vi "get 2d spectrum data.vi"(6 "data in":T5={"Total counts"=0, "cps"=0.0, "live time"=0.0, "pulser"=0.0, "rare counts"=0.0, "other counts"=0.0, "total run time(sec)"=0.0, "adjusted run time(sec)"=0.0, "17O average"=1.0, "17O current"=1.0}, 7 "Cluster":T2, 8 "error in":errorcluster, 9 "number of gated regions":i32=1, 10 "time in":u32, 11 "display array in":T3(array[cluster])) -> (0 "error out":errorcluster, 1 "display array out":T3(array[cluster]), 2 "data out":T5={"Total counts"=0, "cps"=0.0, "live time"=0.0, "pulser"=0.0, "rare counts"=0.0, "other counts"=0.0, "total run time(sec)"=0.0, "adjusted run time(sec)"=0.0, "17O average"=1.0, "17O current"=1.0}, 3 "MCA Histograms":u32[](graph), 4 "channel 0-4 time out":u16[][](array[numeric]), 5 "counts":u32)   [LabVIEW 2016]
doc: "gathers 1d spectrum data for further analysis"
uses:
  controls/count control.ctl
  pixie2d/controls/1d gate selection.ctl
  pixie2d/collectdata Folder/realtime data/pixie vis/controls/number of modules.ctl
panel:
  out "run stats":T4
  out "zero values?":bool
  out "adjusted run time":dbl
  out "total run time":dbl
  out "live time":dbl
  out "cps":dbl
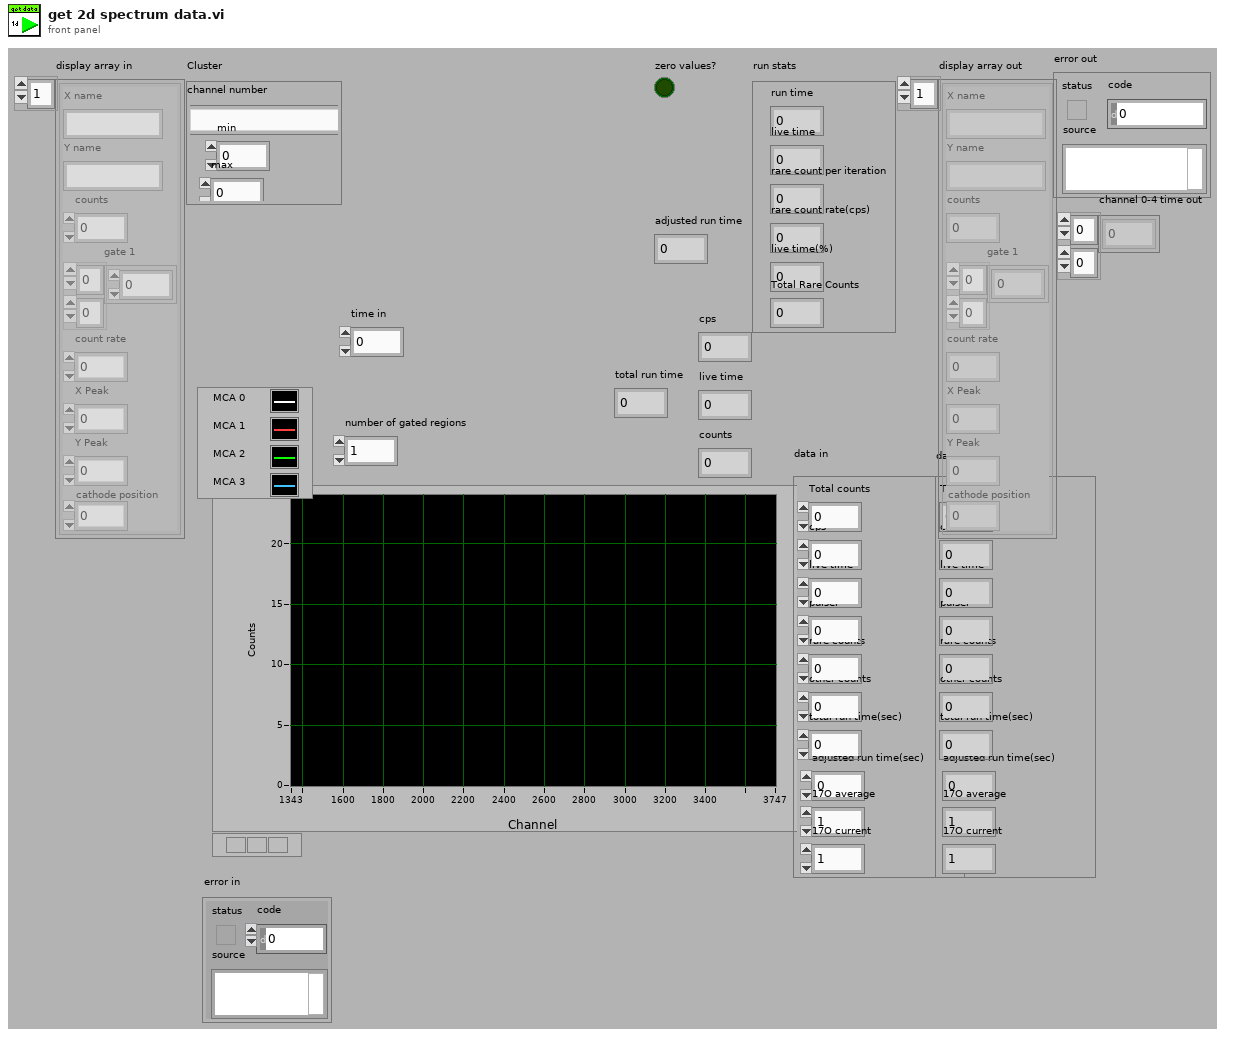
[diagram p1: front panel]
types:
  T1 = typedef "1d gate selection.ctl" = string
  T2 = cluster{"channel number":T1, "min":dbl, "max":dbl}
  T3 = cluster{"X name":string, "Y name ":string, "counts":dbl, "gate 1":dbl[][], "count rate":dbl, "X Peak":dbl, "Y Peak":dbl, "cathode position":dbl}[]
  T4 = cluster{"run time":dbl, "live time":dbl, "rare count per iteration":dbl, "rare count rate(cps)":dbl, "live time(%)":dbl, "Total Rare Counts":dbl}
  T5 = typedef "count control.ctl" = cluster{"Total counts":u32, "cps":dbl, "live time":dbl, "pulser":dbl, "rare counts":dbl, "other counts":dbl, "total run time(sec)":dbl, "adjusted run time(sec)":dbl, "17O average":dbl, "17O current":dbl}
  T6 = typedef "number of modules.ctl" = string
  T7 = cluster{"X name":string, "Y name ":string, "counts":dbl, "gate 1":dbl[][], "count rate":dbl, "X Peak":dbl, "Y Peak":dbl, "cathode position":dbl}
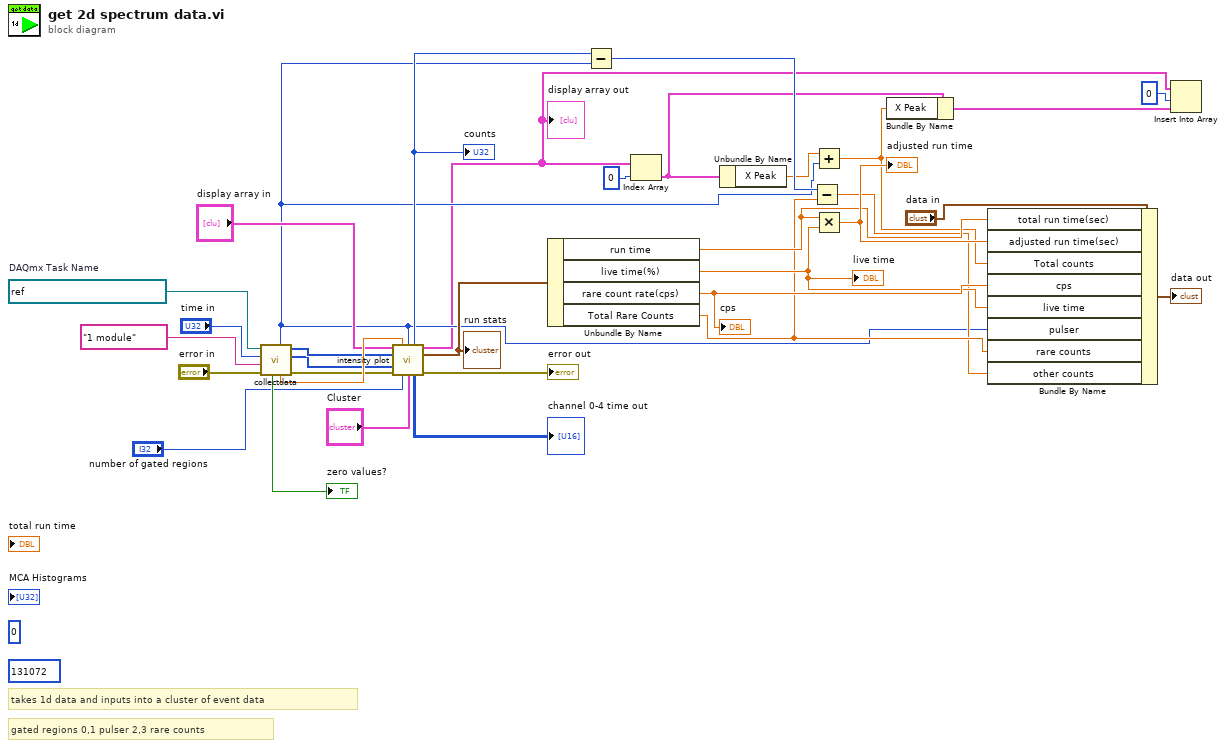
[diagram p0: block diagram]
diagram:
  w31 = refnum<k21> "MyCountEdgesTask"  # DAQmx Task Name
  (unwired) 131072
  (unwired) 0
  # "takes 1d data and inputs into a cluster of event data"
  # "gated regions 0,1 pulser 2,3 rare counts"
  n1 = call "collectdata.vi"("error IO"="error in", "Number of modules"=T6 "1 module", "millisecond timer value"="time in", "DAQmx Task Name"=w31) -> ("error out"=w17:errorcluster, "mod2"=w3:u16[], "listmodedata"=w26:u16[], "labview time"=w27:dbl, "pulses recieved"=w9:u32, "zero values?"=→"zero values?":bool)  [unwired: 1 in, 1 out]
  n2 = call "intensity plot.vi"("display array in"="display array in", "labview time"=w27, "pulses recieved"=w9, "listmodedata in"=w26, "mod 2"=w3, "error IO"=w17, "number of gated regions"="number of gated regions", "Cluster"="Cluster") -> ("Sum of gated counts"=w19:i32, "display array out"=w4:T3, "run stats"=w25:T4, "channel 0-4 time out"=→"channel 0-4 time out":u16[][], "error out"=→"error out":errorcluster)  [unwired: 3 in]
  "counts" <- w19
  "run stats" <- w25
  "display array out" <- w4
  n3 = Unbundle By Name(w25) -> ("run time"=w24:dbl, "live time(%)"=w22:dbl, "rare count rate(cps)"=w23:dbl, "Total Rare Counts"=w21:dbl)
  "cps" <- w23
  "live time" <- w22
  n4 = Subtract(x=w19, y=w9) -> (x-y=w20:u32)
  n5 = Index Array(array=w4, index=0) -> (element=w7:T7)
  n6 = Unbundle By Name(w7) -> ("X Peak"=w10:dbl)
  n7 = Subtract(x=w20, y=w21) -> (x-y=w18:dbl)
  n8 = Add(x=w10, y=w9) -> (x+y=w5:dbl)
  n9 = Multiply(x=w24, y=w22) -> (x*y=w33:dbl)
  "adjusted run time" <- w33
  n10 = Bundle By Name(cluster=w7, "X Peak"=w5) -> (w6:T7)
  n11 = Bundle By Name(cluster="data in", "total run time(sec)"=w24, "adjusted run time(sec)"=w33, "Total counts"=w5, "cps"=w23, "live time"=w22, "pulser"=w9, "rare counts"=w21, "other counts"=w18) -> (→"data out":T5)
  n12 = Insert Into Array(array=w4, index=0, new element=w6) -> ()  [unwired: 1 out]
